vi "ITSERP-Automation-LaunchConfigDialog.vi"() -> ()   [LabVIEW 2013]
panel:
  out "error out":errorcluster
  in  "error in":errorcluster
  out "x = y?":bool
  out "Loading....":u8(slide) scale=0.0..30.0
  out "Loading ITS ERP System":dbl(knob) scale=0.0..4.0
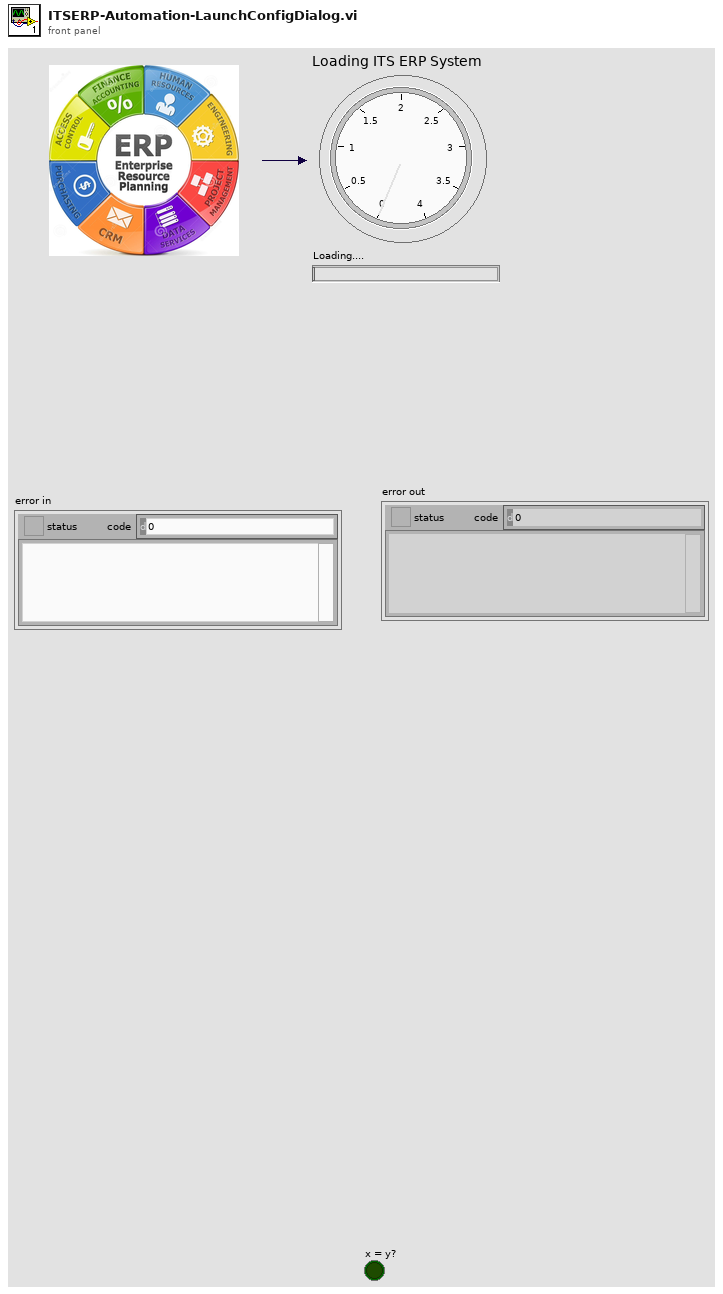
[diagram p1: front panel]
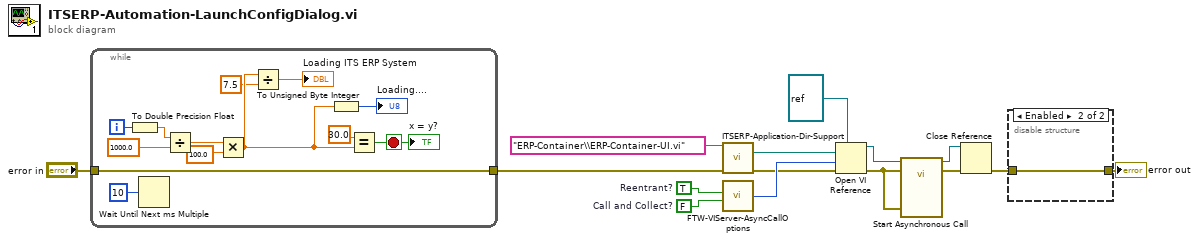
[diagram p0: block diagram]
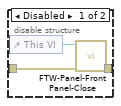
[diagram p2: hidden frame]
diagram:
  w12 = FALSE  # Call and Collect?
  w13 = TRUE  # Reentrant?
  n1 = while {
    tunnel: "error in" -> [w22]
    tunnel: [w22] -> w14
    i -> [w21]
    stop <- w25 stop-if-true
    n2 = To Double Precision Float(number=w21) -> (double precision float=w20:dbl)
    n3 = Wait Until Next ms Multiple(millisecond multiple=u32 10 ("milliseconds to wait")) -> ()  [unwired: 1 out]
    n4 = Divide(x=w20, y=1000.0) -> (x/y=w23:dbl)
    n5 = Multiply(x=w23, y=100.0) -> (x*y=w19:dbl)
    n6 = Divide(x=w19, y=7.5) -> (x/y=→"Loading ITS ERP System":dbl)
    n7 = To Unsigned Byte Integer(number=w19) -> (unsigned 8bit integer=→"Loading....":u8)
    n8 = Equal?(x=30.0, y=w19) -> (x = y?=w25:bool)
    "x = y?" <- w25
  }
  n9 = call "ITSERP-Application-Dir-Support.vi"("Support Resource Relative Filepath"="ERP-Container\\ERP-Container-UI.vi" ("Support VI Relative Filepath"), "error in"=w14) -> ("appended path 2"=w10:path, "error out"=w7:errorcluster)  [unwired: 11 in, 1 out]
  n10 = call "FTW-VIServer-AsyncCallOptions.vi"("Call and Collect?"=w12, "Reentrant?"=w13) -> ("Open VI Ref Options"=w11:i32)  [unwired: 4 in]
  n11 = Open VI Reference(type specifier VI Refnum (for type only)=refnum<vi> refnum, vi path=w10, options=w11, error in (no error)=w7) -> (vi reference=w4:refnum<vi>, error out=w3:errorcluster)  [unwired: 2 in]
  n12 = call-by-ref "Start Asynchronous Call"(reference=w4, error in=w3, "error constant"=w3) -> (reference out=w1:refnum<vi>, error out=w2:errorcluster)  [unwired: 14 in, 1 out]
  n13 = Close Reference(reference=w1, error in (no error)=w2) -> (error out=w8:errorcluster)
  n14 = disable-structure shown="Enabled" {
    disable-tunnel: w8 -> [w31 w32]
    disable-tunnel: [w29 w32] -> w5
    frame Disabled {
      n15 = control-ref of="This VI"() -> (w30:refnum<vi>)
      n16 = call "FTW-Panel-FrontPanel-Close.vi"("error in"=w31, "VI Ref"=w30) -> ("error out"=w29:errorcluster)  [unwired: 8 in, 1 out]
    }
    frame Enabled {
    }
  }
  "error out" <- w5
